vi "CloseSerial.vi"() -> ()   [LabVIEW 2017]
uses:
  <vilib>/Instr/_visa.llb/VISA Configure Serial Port (Instr).vi
panel:
  out "read buffer":string
  in  "VISA resource name":refnum<visa-resource-name>
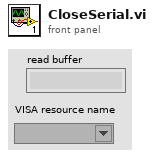
[diagram p1: front panel]
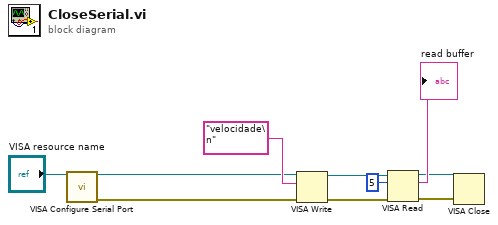
[diagram p0: block diagram]
diagram:
  n1 = call-poly "VISA Configure Serial Port"("VISA resource name"="VISA resource name") -> ("VISA resource name out"=w8:refnum<visa-resource-name>, "error out"=w7:errorcluster)  [unwired: 13 in]
  n2 = VISA Write(VISA resource name=w8, write buffer="velocidade\n", error in (no error)=w7) -> (VISA resource name out=w6:refnum<visa-resource-name>, error out=w5:errorcluster)  [unwired: 1 out]
  n3 = VISA Read(VISA resource name=w6, byte count=u32 5, error in (no error)=w5) -> (VISA resource name out=w2:refnum<visa-resource-name>, read buffer=→"read buffer":string, error out=w1:errorcluster)  [unwired: 1 out]
  n4 = VISA Close(VISA resource name=w2, error in (no error)=w1) -> ()  [unwired: 1 out]
